vi "ConstructorString.vi"(6 "error in":errorcluster, 9 "Control Terminal in":refnum<class "ControlTerminal.lvclass">) -> (0 "error out":errorcluster, 3 "Control Terminal out":refnum<class "ControlTerminal.lvclass">, 4 "constructor":string)   [LabVIEW 2014, in "ControlTerminal.lvclass"]
uses:
  ControlTerminal.lvclass
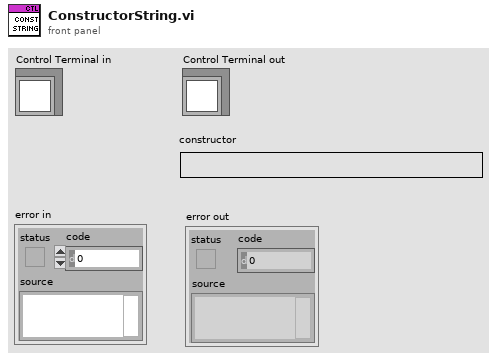
[diagram p1: front panel]
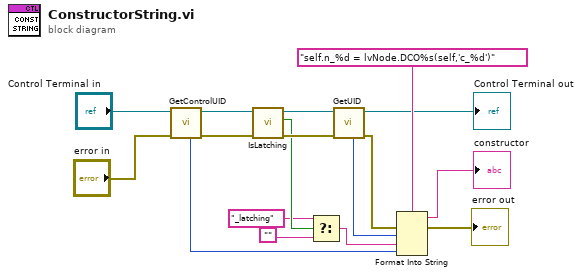
[diagram p0: block diagram]
diagram:
  n1 = call "GetControlUID.vi"("error in"="error in", "Control Terminal in"="Control Terminal in") -> ("error out"=w5:errorcluster, "Control Terminal out"=w6:refnum<class "ControlTerminal.lvclass">, "control UID"=w15:i32)  [unwired: 5 in]
  n2 = call "IsLatching.vi"("error in"=w5, "Control Terminal in"=w6) -> ("error out"=w11:errorcluster, "latching"=w10:bool, "Control Terminal out"=w12:refnum<class "ControlTerminal.lvclass">)  [unwired: 7 in]
  n3 = Select(t="_latching", s=w10, f="") -> (s? t:f=w8:string)
  n4 = call-dynamic "GetUID.vi"("error in"=w11, "GObject in"=w12) -> ("error out"=w3:errorcluster, "GObject out"=→"Control Terminal out":refnum<class "ControlTerminal.lvclass">, "UID"=w13:i32)  [unwired: 5 in]
  n5 = Format Into String(format string="self.n_%d = lvNode.DCO%s(self,'c_%d')", error in=w3, w13, w8, w15) -> (resulting string=→"constructor":string, error out=→"error out":errorcluster)  [unwired: 1 in]
